vi "直方图.vi"() -> ()   [LabVIEW 2018]
uses:
  <vilib>/Analysis/NI_AALPro.lvlib
panel:
  out "第几次":i32
  out "Histogram":i32[](array[numeric]) caption="直方图"
  out "Histogram Graph":T1(graph) caption="直方图"
  in  "# bins":i32 caption="区间数量"
  in  "min":dbl caption="最小值" format="%0.2f"
  in  "max":dbl caption="最大值" format="%0.2f"
  in  "停止":bool
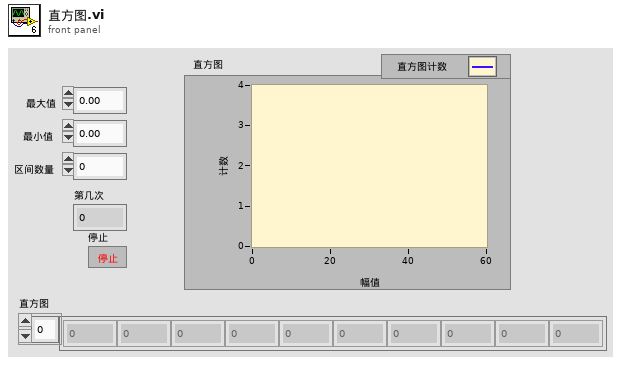
[diagram p1: front panel]
types:
  T1 = cluster{"X Values":dbl[], "Histogram: h(x)":i32[]}
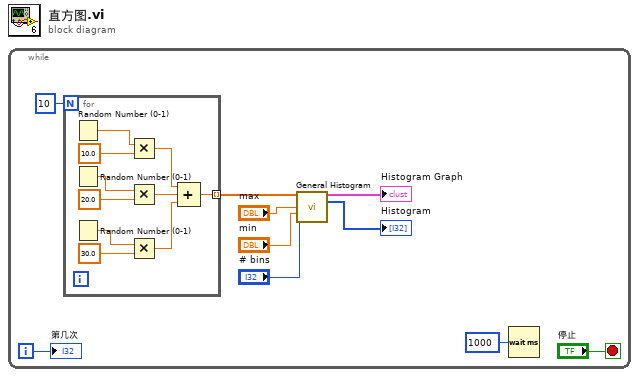
[diagram p0: block diagram]
diagram:
  n1 = while {
    i -> [w1]
    stop <- "停止" stop-if-true
    n2 = for {
      N: 10 -> [_]
      tunnel: [w11] -> w7 mode=indexing
      n3 = Random Number (0-1)() -> (number: 0 to 1=w20:dbl)
      n4 = Random Number (0-1)() -> (number: 0 to 1=w18:dbl)
      n5 = Random Number (0-1)() -> (number: 0 to 1=w16:dbl)
      n6 = Multiply(x=w20, y=10.0) -> (x*y=w14:dbl)
      n7 = Multiply(x=w18, y=20.0) -> (x*y=w13:dbl)
      n8 = Multiply(x=w16, y=30.0) -> (x*y=w12:dbl)
      n9 = Compound Arithmetic op=ADD(w14, w13, w12) -> (w11:dbl)
    }
    n10 = call <vilib>:"General Histogram.vi"("X"=w7, "max"="max", "min"="min", "# bins"="# bins") -> ("Histogram Graph"=→"Histogram Graph":T1, "Histogram"=→"Histogram":i32[])  [unwired: 7 in, 3 out]
    n11 = Wait (ms)(milliseconds to wait=u32 1000 ("等待时间（毫秒）")) -> ()  [unwired: 1 out]
    "第几次" <- w1
  }
